vi "Dashboard Main.vi"() -> ()   [LabVIEW 2015]
uses:
  United/Robot Type Def.ctl
  <vilib>/Rock Robotics/WPI/Camera/WPI_CameraWhite Balance Values.ctl
  <vilib>/Rock Robotics/WPI/Camera/WPI_CameraExposure Values.ctl
  <vilib>/Utility/miscctls.llb/LVRowAndColumnTypeDef.ctl
  <vilib>/event_ctls.llb/eventvkey.ctl
  <vilib>/Rock Robotics/WPI/Dashboard/WPI_DashboardLogging Global.vi
  <vilib>/Rock Robotics/Network Tables/NT Read Numeric Array.vi
  <vilib>/Utility/config.llb/Write Key (String).vi
  <vilib>/Utility/config.llb/Write Key (I32).vi
  <vilib>/Utility/config.llb/NI_LVConfig.lvlib
panel:
  in  "5190Settings":refnum<vi>[][](array[refnum])
  in  "TCP":refnum<k5>
  in  "Rec Mode":enum32{"Stop", "Record", "Playback"}(radio)
  in  "Vision":u16(ring) items=["Camera Off", "USB Camera SW", "USB Camera HW", "IP Camera"]
  out "Camera IP":string
  out "Image Message":string="Timeout in Camera Communications"
  in  "Dashboard Tab":T1(tab)
  in  "Select Auto":string(combo)
  out "NT Connection":bool
  in  "Camera Settings":T2={"Frame Rate"=30, "Compression"=30, "Size"=1} {"Frame Rate" scale=1.0..30.0; "Size" items=["640x480", "320x240", "160x120"]}
  out "MotorChart R":cluster{"Numeric":dbl, "Numeric":dbl}(graph)
  out "MotorChart L":T3(graph)
  out "MotorSliders R":cluster{"MotorSlide1":dbl, "MotorSlide2":dbl} {"MotorSlide2" scale=-1.0..1.0 scale format="%#_2e"; "MotorSlide1" scale=-1.0..1.0 scale format="%#_2e"}
  out "MotorSliders L":T4 {"MotorSlide4 2" scale=0.0..14.0 scale format="%#_2e"; "MotorSlide2" scale=-1.0..1.0 scale format="%#_2e"; "MotorSlide1" scale=-1.0..1.0 scale format="%#_2e"}
  out "Gyro":dbl(knob) scale=0.0..360.0
  out "JS1 Z":dbl(slide) scale=-1.0..1.0 scale format="%#_2e"
  out "JS1 Graph":cluster{"X":dbl, "Y":dbl}[](graph)
  out "JS1 Buttons":T5
  out "JS2 Z":dbl(slide) scale=-1.0..1.0 scale format="%#_2e"
  out "JS2 Graph":cluster{"X":dbl, "Y":dbl}[](graph)
  out "JS2 Buttons":T5
  out "Mode":T6(ring)=enum."Auto Disabled"
  in  "DB Camera Config":bool
  out "fps":dbl format="%#.1g"
  out "Mbps":dbl format="%#.1g"
  out "Mbps LED":bool
  in  "Test Slider":dbl(slide) scale=0.0..100.0 scale format="%#_3g"
  in  "On/Off":bool caption="Solenoid"
  in  "Test Name":u16(ring) items=["Select the test to run..."]
  in  "Test Tree":string(tree)
  in  "Motor":cluster{"Value":dbl, "Enable":bool} {"Value" scale=-1.0..1.0 scale format="%#_3g"}
  out "Progress":T7 {"Test Progress" scale=0.0..100.0}
  in  "Rev/Fwd":cluster{"Forward":bool, "Reverse":bool}
  in  "Test Ring":u16(ring) items=["Monochrome", "Color"]
  out "Cmd Status":string
  in  "Execute Command":bool
  in  "Command Params":string[][](table)
  in  "Command Selection":i32(listbox)
  in  "CheckList":i32(listbox)
  out "Tree":string(tree)
  in  "Tab Control":T8(tab)
  in  "Joystick Deadband":dbl format="%#_13g"
  out "Sent":bool
  in  "Send Values to Robot":bool
  in  "Robot":T9
  in  "AutoPlaySelect":T10(ring)=enum."Play02"
  in  "EncTics5":dbl
  in  "updistance":dbl
  in  "Radius":dbl
  in  "R5":dbl
  in  "IZ5":dbl
  in  "F5":dbl
  in  "D5":dbl
  in  "I5":dbl
  in  "P5":dbl
  in  "Turn Damp":dbl format="%#_13g"
  in  "P 2":dbl format="%#_13g"
  in  "I 2":dbl format="%#_13g"
  in  "D 2":dbl format="%#_13g"
  in  "F 2":dbl format="%#_13g"
  in  "R 2":dbl format="%#_13g"
  in  "IZ 2":dbl format="%#_13g"
  in  "P":dbl format="%#_13g"
  in  "I":dbl format="%#_13g"
  in  "D":dbl format="%#_13g"
  in  "R":dbl format="%#_13g"
  in  "F":dbl format="%#_13g"
  in  "IZ":dbl format="%#_13g"
  in  "EncTicsPerRev":dbl format="%#_13g"
  in  "ClimberRevs":dbl
  in  "P 3":dbl format="%#_13g"
  in  "IZ 3":dbl format="%#_13g"
  in  "R 3":dbl format="%#_13g"
  in  "I 3":dbl format="%#_13g"
  in  "F 3":dbl format="%#_13g"
  in  "D 3":dbl format="%#_13g"
  in  "Up Angle(Ticks)":dbl format="%#_13g"
  in  "EncTicsPerRev 2":dbl format="%#_13g"
  in  "Down Angle(Ticks)":dbl format="%#_13g"
  in  "Shoot Delay":dbl
  in  "Shoot Continue":dbl
  in  "Intake Close Claw":dbl
  in  "Intake Time Limit":dbl
  in  "DeltaAngle":dbl
  in  "TopOutSpeed":dbl
  in  "BottomOutSpeed":dbl
  in  "TopInSpeed":dbl
  in  "BottomInSpeed":dbl
  in  "P 4":dbl format="%#_13g"
  in  "IZ 4":dbl format="%#_13g"
  in  "R 4":dbl format="%#_13g"
  in  "I 4":dbl format="%#_13g"
  in  "F 4":dbl format="%#_13g"
  in  "D 4":dbl format="%#_13g"
  in  "EncTicsPerRev 3":dbl format="%#_13g"
  in  "Brightness":dbl
  in  "Compression":dbl
  in  "Exposure":T11=enum."Flicker-free 60 Hz"
  in  "White Balance":T12=enum."Fixed indoor"
  in  "FPS":dbl
  in  "Masked":bool
  in  "LED Color":T13={"Hue"={110.52399131877658, 148.6727294921875}, "Sat"={34.78571428571429, 255.0}, "Val"={91.07142857142858, 255.0}} {"Hue" scale=0.0..255.0 scale format="%#_3g"}
  out "X Deg":dbl
  out "Y Deg":dbl
  in  "LapTop Cam":bool
  out "Camera Image":T14(plugin-control)
  out "Background":bool
  # "Left"
  # "Front"
  # "Right"
  # "Battery"
  # "Autonomous Mode Save File: /home/lvuser/Autonomous/Play/Play##.csv\nCommands:\nTime:\n    0   MS       0      0\n\nStraight:\n    1   INCHES   0      0 \n\nTurn:\n    2   ANGLE    SPEED  0   \n \nArm Set Angle:\n    3   ANGLE    0      0 \n\nShoot:\n    4   0              0            0"
  # "PID for the Tape"
  # "All Units in Inches"
  # "Distance"
  # "Speed"
  # "Postion"
  # "Roller Speeds"
  # "Shooter ARM PID"
  # "Solenoid Delays"
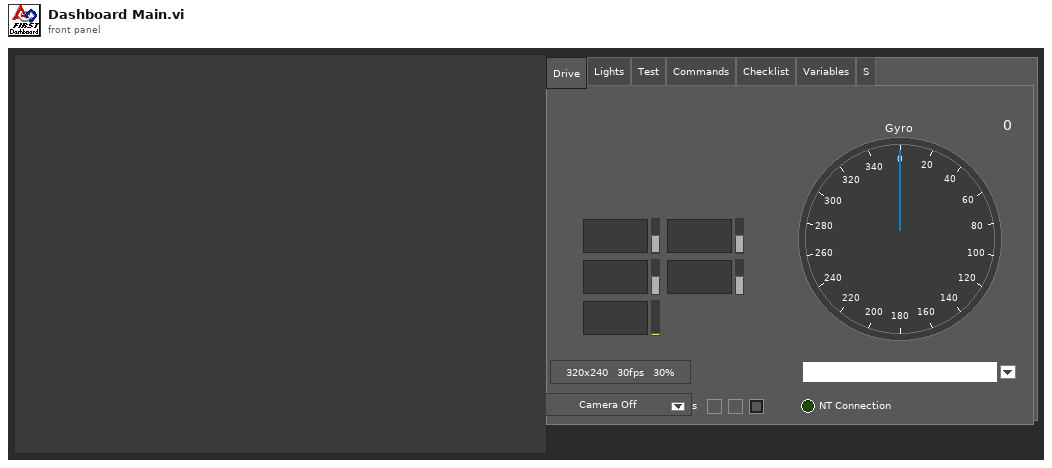
[diagram p1: front panel]
types:
  T1 = enum32{"Drive", "Lights", "Test", "Commands", "Checklist", "Variables", "S"}
  T2 = cluster{"Frame Rate":i32, "Compression":i32, "Size":u16}
  T3 = cluster{"Numeric":dbl, "Numeric":dbl, "Battery V":dbl}
  T4 = cluster{"MotorSlide1":dbl, "MotorSlide2":dbl, "MotorSlide4 2":dbl}
  T5 = cluster{bool, bool, bool, bool, bool, bool, bool, bool, bool, bool, bool, bool}
  T6 = enum8{"Tele-Op Disabled", "Tele-Op Enabled", "Auto Disabled", "Auto Enabled", "Test Disabled", "Test Enabled", "Disconnected", "No Code", "E-Stop"}
  T7 = cluster{"Test Progress":u8, "Test Progress Text":string}
  T8 = enum32{"Main", "Auto", "Tape", "Drive", "Port C", "Shooter", "Vision"}
  T9 = typedef "Robot Type Def.ctl" = enum32{"Disabled", "Ghost", "Casper", "Lofty", "Board", "RaceRobot"}
  T10 = enum16{"Play00", "Play01", "Play02", "Play03", "Play04", "Play05"}
  T11 = typedef "WPI_CameraExposure Values.ctl" = enum16{"Auto", "Flicker-free 50 Hz", "Flicker-free 60 Hz", "Hold current", "Custom"}
  T12 = typedef "WPI_CameraWhite Balance Values.ctl" = enum16{"Auto", "Fixed indoor", "Fixed outdoor 1", "Fixed outdoor 2", "Fixed fluorescent 1", "Fixed fluorescent 2", "Hold current", "Custom"}
  T13 = cluster{"Hue":cluster{dbl, dbl}, "Sat":cluster{dbl, dbl}, "Val":cluster{dbl, dbl}}
  T14 = typedef "IMAQ Image.ctl" = refnum<image>
  T15 = typedef "Image Type" = u32
  T16 = cluster{"IDs":cluster{"RPC field ID":u16, "Unique ID":u16}, "String":string}
  T17 = enum32{"Drive", "Lights", "Test", "Commands", "Checklist", "Variables"}
  T18 = enum32{"Drive", "Basic", "Custom", "Test", "Checklist", "Variables"}
  T19 = cluster{"Camera Image":refnum<vi>, "Dashboard Tab":refnum<vi>, "Background":refnum<vi>, "Vision":refnum<vi>, "Rec Mode":refnum<vi>, "Test Slider":refnum<vi>, "On/Off ":refnum<vi>, "Test Ring":refnum<vi>, "Rev/Fwd":refnum<vi>, "Test Name":refnum<vi>, "Motor":refnum<vi>, "Progress":refnum<vi>, "CheckList":refnum<vi>, "Tree":refnum<vi>, "Test Tree":refnum<vi>, "Command Params":refnum<vi>, "Command Selection":refnum<vi>, "Execute Command":refnum<vi>, "Cmd Status":refnum<vi>}
  T20 = cluster{"Error Strings":string, "Disable Counts":cluster{u16, u16}, "Rail Faults":cluster{u16, u16, u16}, "Robot IP":string, "DB Mode":u8, "Event Info":cluster{"Name":string, "Type":u8, "Number":u16, "Replay":u8}, "Camera Addr":string}
  T21 = cluster{"Storage":cluster{"Disk Free":u64, "RAM Block":u32, "RAM free":u32}, "CPU Utilization":cluster{"CPU % ISR":sgl, "CPU % Time Crit":sgl, "CPU % Timed Str":sgl, "CPU % High":sgl, "CPU % Above":sgl, "CPU % Normal":sgl, "CPU % Low":sgl}, "CAN":cluster{"% Bus Utilization":sgl, "Bus Off Cnt":u32, "TX_FIFO Full Cnt":u32, "Receive Error Cnt":u8, "Transmit Error Cnt":u8}, "HID":cluster{"HID Outputs":u32, "Rumble Low":u16, "Rumble High":u16}[]}
  T22 = cluster{"Status bits":cluster{"Test Mode":bool, "Autonomous":bool, "Enabled":bool, "Code Start":bool, "Brownout":bool, "Reserved 2":bool, "Reserved 3":bool, "E-Stop":bool}, "Code Trace":cluster{"Disabled":bool, "TeleOp":bool, "Auto":bool, "Test":bool}, "Controller Type":enum16{"unknown", "cRIO", "roboRio"}, "Code?":enum16{"unknown", "noCode", "code"}, "Battery V":dbl}
  T23 = cluster{"Control Bits":cluster{"TestMode":bool, "Autonomous":bool, "Enabled":bool, "FMS Present":bool, bool, bool, bool, "E-Stop":bool}, "Team Station ":u8, "Countdown":sgl, "Joystick Values":cluster{"Axes":dbl[], "Buttons":bool[], "POVs":i16[]}[]}
  T24 = cluster{"Axes":dbl[], "Buttons":bool[], "POVs":i16[]}[]
  T25 = cluster{"Axes":dbl[], "Buttons":bool[], "POVs":i16[]}
  T26 = cluster{"Buttons[0]":bool, "Buttons[1]":bool, "Buttons[2]":bool, "Buttons[3]":bool, "Buttons[4]":bool, "Buttons[5]":bool, "Buttons[6]":bool, "Buttons[7]":bool, "Buttons[8]":bool, "Buttons[9]":bool, "Buttons[10]":bool, "Buttons[11]":bool}
  T27 = typedef "NI_LVConfig.lvlib/Config Data RefNum.ctl" = refnum<k1>
  T28 = cluster{"Operation":enum16{"Update", "Clear"}, "Color Box":u32}[]
  T29 = typedef "eventvkey.ctl" = enum16{"ASCII", "Enter", "Return", "Shift", "Ctrl", "Alt", "Cmd", "Opt", "Caps", "NumLock", "Clear", "Break", "Up", "Down", "Left", "Right", "Insert", "Delete", "Home", "End", "PageUp", "PageDown", "Escape", "Help", "Pause", "ScrollLock", "F1", "F2", "F3", "F4", "F5", "F6", "F7", "F8", "F9", "F10", "F11", "F12", "F13", "F14", "F15", "F16", "F17", "F18", "F19", "F20", "F21", "F22", "F23", "F24", "Play", "VolumeUp", "VolumeDown", "Mute", "Two Byte Char"}
  T30 = cluster{"Image Size":bool, "Image Type":bool, "Pixel Value":bool, "ROI Information":bool, "Zoom Factor":bool}
  T31 = enum8{"Enabled", "Disabled", "Disabled and Grayed Out"}
  T32 = cluster{"Operation":enum16{"Update", "Clear"}, "Color Box":u32}
  T33 = typedef "LVRowAndColumnTypeDef.ctl" = cluster{"Row":i32, "Column":i32}
  T34 = cluster{"Shift":bool, "Ctrl":bool, "Alt":bool, "Cmd":bool, "Opt":bool}
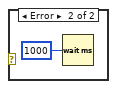
[diagram p2: hidden frame]
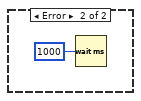
[diagram p3: hidden frame]
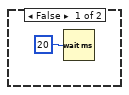
[diagram p4: hidden frame]
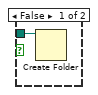
[diagram p6: hidden frame]
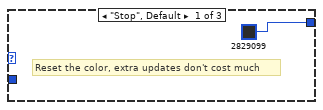
[diagram p7: hidden frame]
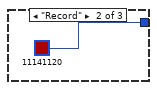
[diagram p8: hidden frame]
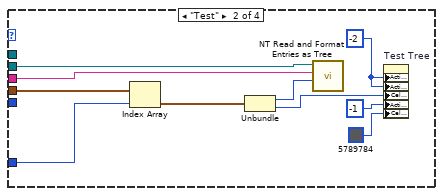
[diagram p10: hidden frame]
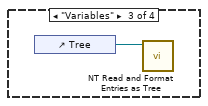
[diagram p11: hidden frame]
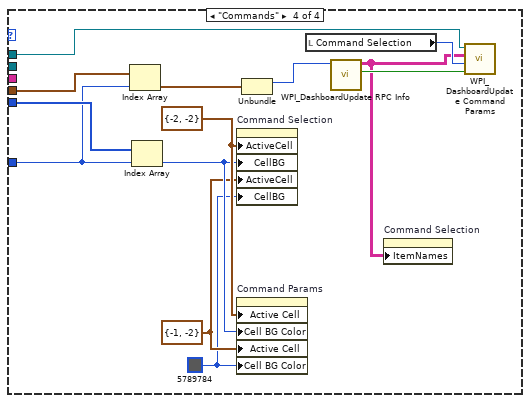
[diagram p12: hidden frame]
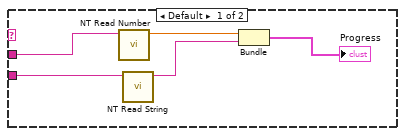
[diagram p13: hidden frame]
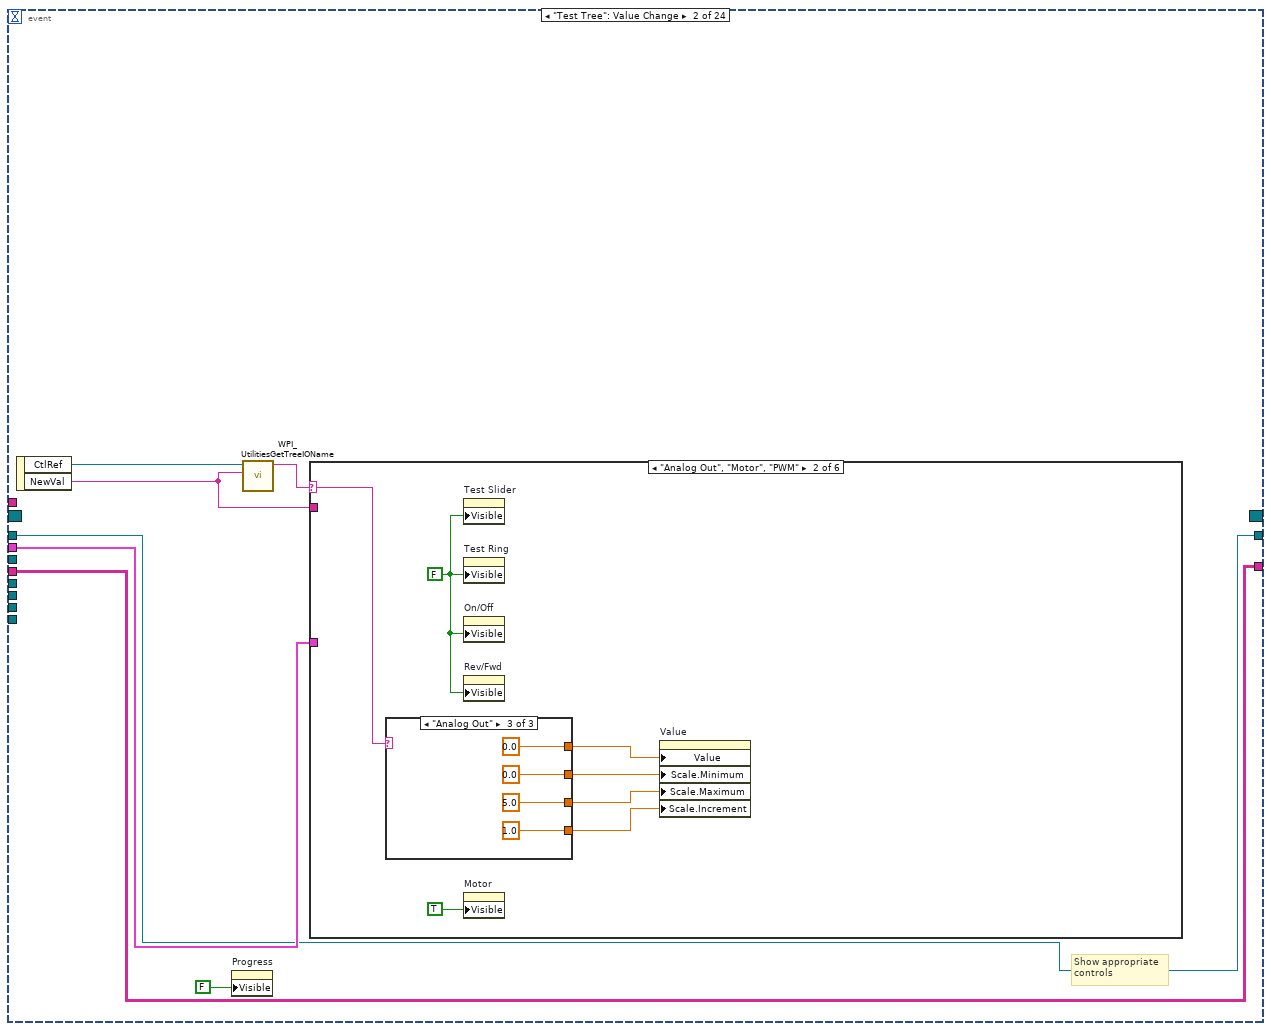
[diagram p14: hidden frame]
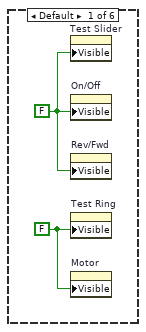
[diagram p15: hidden frame]
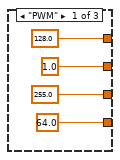
[diagram p16: hidden frame]
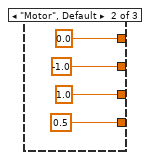
[diagram p17: hidden frame]
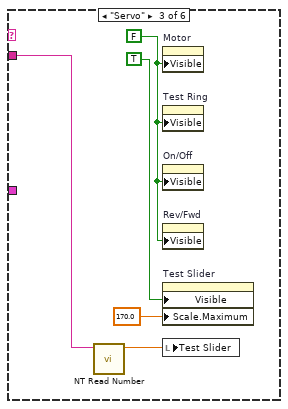
[diagram p18: hidden frame]
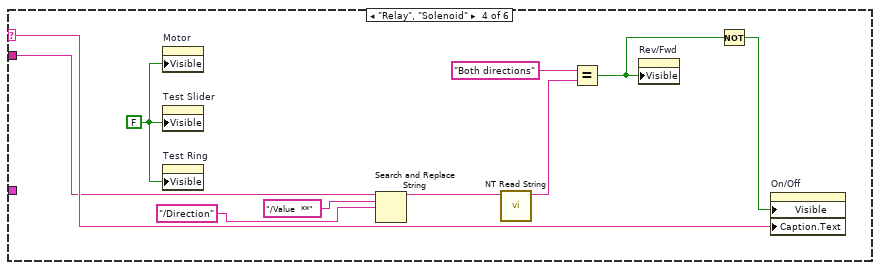
[diagram p19: hidden frame]
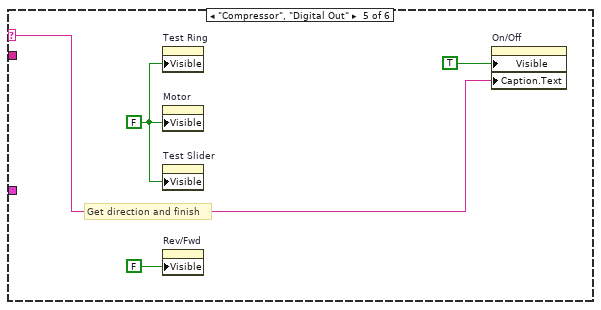
[diagram p20: hidden frame]
diagram:
  w67 = T15 4 items=["Grayscale (U8)", "Grayscale (I16)", "Grayscale (SGL)", "Complex (CSG)", "RGB (U32)", "HSL (U32)", "RGB (U64)", "Grayscale (U16)"] ("Image Type")
  w75 = T16 {"IDs"={"RPC field ID"=0, "Unique ID"=0}, "String"=""}  # RPC Response
  w100 = 491  # min tab size
  w99 = 1.333  # min tab size
  w108 = enum32{"Stop", "Record", "Playback"}."Stop" ("Rec Mode")
  w82 = FALSE ("Visible")
  w128 = T15 4 items=["Grayscale (U8)", "Grayscale (I16)", "Grayscale (SGL)", "Complex (CSG)", "RGB (U32)", "HSL (U32)", "RGB (U64)"] ("Image Type")
  # "Low Shooter\nIndex 3"
  # "Tape \nIndex 5"
  # "Ghost uses Durations and Speeds for In/Out\nCasper uses switches for that"
  # "PortC\nIndex 2"
  # "DriveTrain\nIndex-1"
  # "Robot Type and AutoPlay\nIndex 0"
  # "S"
  # "Open file and read it Once and Only Once"
  # "Command Param Info"
  # "Started one, Unique ID holds\nresponse"
  # "Loop 7. Wait for DS connections"
  # "Basic debug and auto controls: Their data names are fixed, but\nthe displayed name, called a caption, can be changed directly or in\nrobot code such as shown in Begin."
  # "Controls for Test Mode, Camera Settings, etc."
  # "Additional UI Initialization"
  # "Loop 6. Animation for background of window during playback and record"
  # "Fires each time robot IP\nchanges, simulator does this"
  # "Fires each time window\ndocking changes."
  # "Collects all controls and indicators\nin the Basic and Custom tab.\nIf you need to bind additional controls,\nadd their references. You can extend the\nenum constant or use an integer."
  # "The remaining code below this line typically doesn't need to be modified."
  # "Loop 4. Process UI events related to test mode, checklist, and camera settings"
  # "Terminals of controls and indicators that are bound to the smart dashboard by name.\nYou can place the terminals anywhere you like and even read data from them.\nYou bind controls by adding the control reference to the array on the left. The subVI will\ndo this for the contents of a tab, and you can do it for individual items too, as shown with\nthe LED. To create get the reference, right-click and Create>>Reference."
  # "Loop 3. Wait until the robot response provides\n the Robot IP address.\nOnce known, bind controls and\nvariables with the same names."
  # "Loop 5. Adjusts placement onscreen, hides the titlebar, etc."
  # "Loop 2. Receive camera images from Robot, update Mbps, fps, and do any processing or display"
  n1 = control-ref of="DeltaAngle"() -> (w64:refnum<vi>)
  n2 = control-ref of="Joystick Deadband"() -> (w1:refnum<vi>)
  n3 = control-ref of="Robot"() -> (w41:refnum<vi>)
  n4 = control-ref of="updistance"() -> (w23:refnum<vi>)
  n5 = control-ref of="BottomOutSpeed"() -> (w54:refnum<vi>)
  n6 = control-ref of="Intake Time Limit"() -> (w21:refnum<vi>)
  n7 = control-ref of="Intake Close Claw"() -> (w20:refnum<vi>)
  n8 = control-ref of="Up Angle(Ticks)"() -> (w4:refnum<vi>)
  n9 = control-ref of="EncTicsPerRev 3"() -> (w63:refnum<vi>)
  n10 = control-ref of="EncTicsPerRev 2"() -> (w3:refnum<vi>)
  n11 = control-ref of="BottomInSpeed"() -> (w52:refnum<vi>)
  n12 = control-ref of="Shoot Continue"() -> (w18:refnum<vi>)
  n13 = control-ref of="AutoPlaySelect"() -> (w42:refnum<vi>)
  n14 = control-ref of="TopOutSpeed"() -> (w55:refnum<vi>)
  n15 = control-ref of="Down Angle(Ticks)"() -> (w2:refnum<vi>)
  n16 = control-ref of="TopInSpeed"() -> (w53:refnum<vi>)
  n17 = control-ref of="Shoot Delay"() -> (w19:refnum<vi>)
  n18 = control-ref of="P 3"() -> (w10:refnum<vi>)
  n19 = control-ref of="I 3"() -> (w9:refnum<vi>)
  n20 = control-ref of="D 3"() -> (w8:refnum<vi>)
  n21 = control-ref of="F 3"() -> (w7:refnum<vi>)
  n22 = control-ref of="IZ 3"() -> (w6:refnum<vi>)
  n23 = control-ref of="R 3"() -> (w5:refnum<vi>)
  n24 = control-ref of="Brightness"() -> (w12:refnum<vi>)
  n25 = control-ref of="Compression"() -> (w13:refnum<vi>)
  n26 = control-ref of="EncTicsPerRev"() -> (w40:refnum<vi>)
  n27 = control-ref of="Exposure"() -> (w14:refnum<vi>)
  n28 = control-ref of="FPS"() -> (w16:refnum<vi>)
  n29 = control-ref of="ClimberRevs"() -> (w48:refnum<vi>)
  n30 = control-ref of="White Balance"() -> (w15:refnum<vi>)
  n31 = control-ref of="Turn Damp"() -> (w32:refnum<vi>)
  n32 = control-ref of="F 2"() -> (w45:refnum<vi>)
  n33 = control-ref of="IZ 2"() -> (w46:refnum<vi>)
  n34 = control-ref of="R 2"() -> (w47:refnum<vi>)
  n35 = Build Array(w10, w9, w8, w7, w6, w5, w3, w2, w4) -> (w58:refnum<vi>[])
  n36 = control-ref of="P"() -> (w33:refnum<vi>)
  n37 = control-ref of="I"() -> (w34:refnum<vi>)
  n38 = control-ref of="D"() -> (w35:refnum<vi>)
  n39 = control-ref of="F"() -> (w36:refnum<vi>)
  n40 = control-ref of="IZ"() -> (w43:refnum<vi>)
  n41 = control-ref of="R"() -> (w44:refnum<vi>)
  n42 = control-ref of="P 2"() -> (w37:refnum<vi>)
  n43 = control-ref of="I 2"() -> (w38:refnum<vi>)
  n44 = control-ref of="D 2"() -> (w39:refnum<vi>)
  n45 = control-ref of="P 4"() -> (w49:refnum<vi>)
  n46 = control-ref of="I 4"() -> (w50:refnum<vi>)
  n47 = control-ref of="D 4"() -> (w51:refnum<vi>)
  n48 = control-ref of="F 4"() -> (w60:refnum<vi>)
  n49 = control-ref of="IZ 4"() -> (w61:refnum<vi>)
  n50 = control-ref of="R 4"() -> (w62:refnum<vi>)
  n51 = control-ref of="P5"() -> (w31:refnum<vi>)
  n52 = control-ref of="I5"() -> (w30:refnum<vi>)
  n53 = control-ref of="D5"() -> (w29:refnum<vi>)
  n54 = control-ref of="F5"() -> (w28:refnum<vi>)
  n55 = control-ref of="IZ5"() -> (w27:refnum<vi>)
  n56 = control-ref of="R5"() -> (w26:refnum<vi>)
  n57 = control-ref of="EncTics5"() -> (w25:refnum<vi>)
  n58 = control-ref of="Radius"() -> (w24:refnum<vi>)
  n59 = Build Array(w41, w42, w1) -> (w56:refnum<vi>[])
  n60 = Build Array(w33, w34, w35, w36, w43, w44, w37, w38, w39, w45, w46, w47, w40, w48, w32) -> (w57:refnum<vi>[])
  n61 = Build Array(w49, w50, w51, w60, w61, w62, w63, w52, w53, w54, w55, w64, w21, w20, w19, w18) -> (w59:refnum<vi>[])
  n62 = Build Array(w31, w30, w29, w28, w27, w26, w25, w24, w23) -> (w22:refnum<vi>[])
  n63 = Build Array(w16, w15, w14, w13, w12) -> (w11:refnum<vi>[])
  n64 = Build Array(w56, w57, w58, w59, w22, w11) -> (w17:refnum<vi>[][])
  n65 = local write "5190Settings"(w17) -> ()
  n66 = call "Init.vi"("Array"=w17) -> ()  [unwired: 11 in]
  n67 = Obtain Notifier(name (unnamed)="Robot IP Update", notification data type="IP Addr" ("name (unnamed)")) -> (notifier out=w68:refnum<notifier>)  [unwired: 2 in, 2 out]
  n68 = control-ref of="Rec Mode"() -> (w88:refnum<vi>)
  n69 = control-ref of="Command Selection"() -> (w74:refnum<vi>)
  n70 = control-ref of="Camera Image"() -> (w103:refnum<vi>)
  n71 = control-ref of="Tree"() -> (w92:refnum<vi>)
  n72 = control-ref of="Test Tree"() -> (w91:refnum<vi>)
  n73 = control-ref of="Dashboard Tab"() -> (w102:refnum<vi>)
  n74 = control-ref of="Execute Command"() -> (w76:refnum<vi>)
  n75 = control-ref of="Background"() -> (w97:refnum<vi>)
  n76 = control-ref of="On/Off"() -> (w86:refnum<vi>)
  n77 = control-ref of="Progress"() -> (w83:refnum<vi>)
  n78 = control-ref of="Rev/Fwd"() -> (w84:refnum<vi>)
  n79 = control-ref of="Motor"() -> (w89:refnum<vi>)
  n80 = control-ref of="Cmd Status"() -> (w70:refnum<vi>)
  n81 = control-ref of="Command Params"() -> (w77:refnum<vi>)
  n82 = control-ref of="Test Slider"() -> (w87:refnum<vi>)
  n83 = control-ref of="Vision"() -> (w101:refnum<vi>)
  n84 = control-ref of="Test Ring"() -> (w85:refnum<vi>)
  n85 = control-ref of="Test Name"() -> (w90:refnum<vi>)
  n86 = property class="VI" props=["Front Panel.Closeable"]() -> (reference out=w107:refnum<vi>)  [unwired: 2 in, 2 out]
  n87 = control-ref of="Command Params"() -> (w69:refnum<vi>)
  n88 = control-ref of="CheckList"() -> (w93:refnum<vi>)
  n89 = Bundle("min tab size"=w100, "min tab size"=w99) -> (w98:cluster{"min tab size":i32, "min tab size":dbl})  [unwired: 1 in]
  n90 = Create User Event(user event datatype=w75) -> (user event=w71:refnum<user-event>)  [unwired: 1 in, 1 out]
  n91 = Obtain Notifier(name (unnamed)="Window Mode", notification data type=TRUE) -> (notifier out=w80:refnum<notifier>)  [unwired: 2 in, 2 out]
  n92 = Bundle("Camera Image"=w103, "Dashboard Tab"=w102, "Background"=w97, "Vision"=w101, "Rec Mode"=w88, "Test Slider"=w87, "On/Off"=w86, "Test Ring"=w85, "Rev/Fwd"=w84, "Test Name"=w90, "Motor"=w89, "Progress"=w83, "CheckList"=w93, "Tree"=w92, "Test Tree"=w91, "Command Params"=w77, "Command Selection"=w74, "Execute Command"=w76, "Cmd Status"=w70) -> (w94:T19)  [unwired: 1 in]
  n93 = control-ref of="Dashboard Tab"() -> (w106:refnum<vi>)
  n94 = call "IMAQ Create"("Image Name"="Dashboard Image", "Image Type"=w128) -> ("New Image"=w126:T14, "error out"=w125:errorcluster)  [unwired: 2 in, 1 out]
  n95 = call "IMAQ Create"("Image Name"="LapTop Cam", "Image Type"=w67) -> ("New Image"=w65:T14)  [unwired: 2 in, 2 out]
  n96 = call <vilib>:"Get Tab Control Refs.vi"("Page Index"=T18."Basic" ("Dashboard Tab"), "TabControl in"=w106) -> ("ControlsOnPage"=w81:refnum<vi>[])  [unwired: 9 in]
  n97 = while {
    tunnel: [w142] -> _
    tunnel: w68 -> [w137]
    tunnel: w81 -> [w136]
    tunnel: w80 -> [w132]
    i -> [w142]
    stop <- FALSE stop-if-true
    n98 = call <vilib>:"WPI_DashboardUpdateNames.vi"("Controls on Tab"=w136) -> ()  [unwired: 11 in]
    n99 = local read "Vision"() -> (w134:u16)
    n100 = call <vilib>:"WPI_DashboardRetrieveStatusInfo.vi"("Vision"=w134, "Binding Refnum"=w137, "Window Mode Notifier"=w132, "TCP Cnx"="TCP") -> ("Power and Errors"=w138:T20, "Robot Metrics"=w140:T21, "Status Info"=w141:T22, "Control Info"=w139:T23, "Robot Mode"=w135:T6, "Process?"=w131:bool)  [unwired: 2 in]
    "Mode" <- w135
    n101 = feedback-in #1(w131) -> ()
    n102 = feedback #1(FALSE) -> (w129:bool)
    n103 = case shown="True" w131 {
      tunnel: w141 -> [_ w175]
      tunnel: w140 -> [_ w174]
      tunnel: w139 -> [_ w173]
      tunnel: w138 -> [_ w172]
      tunnel: w135 -> [_ _]
      tunnel: w129 -> [_ w148]
      frame False {
        n104 = Wait (ms)(milliseconds to wait=u32 20) -> ()  [unwired: 1 out]
      }
      frame True {
        # "swap motors to match\ncharts and include battery"
        n105 = Not(x=w148) -> (.not. x?=w146:bool)
        n106 = Unbundle By Name(w173) -> ("Joystick Values"=w162:T24)  [unwired: 1 out]
        n107 = Unbundle By Name(w174) -> ()  [unwired: 1 out]
        n108 = Unbundle By Name(w172) -> ("Camera Addr"=→"Camera IP":string)  [unwired: 1 out]
        n109 = Unbundle By Name(w175) -> ("Battery V"=w163:dbl)  [unwired: 1 out]
        n110 = Or(x="Send Values to Robot", y=w146) -> (x .or. y?=w145:bool)
        n111 = Index Array(array=w162) -> (element #1=w161:T25, element #2=w156:T25)  [unwired: 2 in]
        n112 = case shown="True" w145 {
          frame False {
          }
          frame True {
            n113 = flat-sequence {
              tunnel: [TRUE] -> w176
              frame #0 {
                n114 = local write "Sent"(FALSE) -> ()
              }
              frame #1 {
                w178 = path "C:/5190data" ("path")
                n115 = call <vilib>:"Check if File or Folder Exists.vi"("path"=w178) -> ("file or folder exists?"=w179:bool)  [unwired: 8 in, 2 out]
                n116 = case shown="True" w179 {
                  tunnel: w178 -> [w180 _]
                  frame False {
                    n117 = Create Folder(path (use dialog)=w180) -> ()  [unwired: 2 in, 3 out]
                  }
                  frame True {
                  }
                }
              }
              frame #2 {
                n118 = local read "5190Settings"() -> (w182:refnum<vi>[][])
                n119 = call "Read-Write-Settings.vi"("appended array 4"=w182, "Write"=TRUE) -> ()  [unwired: 5 in, 1 out]
              }
            }
            "Sent" <- w176
          }
        }
        n120 = call-poly <vilib>:"NT Read Value.vi"("Name"="NavX Yaw") -> ("Numeric"=→"Gyro":dbl)  [unwired: 9 in, 1 out]
        n121 = call "Prepare Joystick Data for Displays.vi"("Joystick Values"=w161) -> ("Buttons"=→"JS1 Buttons":T26, "Z Axis"=→"JS1 Z":dbl, "Cartesian Data"=→"JS1 Graph":cluster{"X axis":dbl, "X axis":dbl}[])  [unwired: 8 in]
        n122 = call "Prepare Joystick Data for Displays.vi"("Joystick Values"=w156) -> ("Buttons"=→"JS2 Buttons":T26, "Z Axis"=→"JS2 Z":dbl, "Cartesian Data"=→"JS2 Graph":cluster{"X axis":dbl, "X axis":dbl}[])  [unwired: 8 in]
        n123 = call-poly <vilib>:"NT Read Value.vi"("Name"="RobotDrive Motors") -> ("Numeric Array"=w151:dbl[])  [unwired: 9 in, 1 out]
        n124 = Index Array(array=w151, index #1=1, index #4=0) -> (element #1=w167:dbl, element #2=w168:dbl, element #3=w166:dbl, element #4=w171:dbl)  [unwired: 2 in]
        n125 = Bundle("Numeric"=w166, "Numeric"=w167) -> (→"MotorChart R" →"MotorSliders R":cluster{"Numeric":dbl, "Numeric":dbl})  [unwired: 1 in]
        n126 = Bundle("Numeric"=w168, "Numeric"=w171, "Battery V"=w163) -> (→"MotorChart L" →"MotorSliders L":T3)  [unwired: 1 in]
      }
    }
  }
  n127 = call <vilib>:"Get Tab Control Refs.vi"("Page Index"=T18."Custom" ("Dashboard Tab"), "TabControl in"=w106) -> ("ControlsOnPage"=w105:refnum<vi>[])  [unwired: 9 in]
  n128 = while {
    tunnel: w126 -> [w199]
    tunnel: w125 -> [_]
    tunnel: [w200] -> _
    tunnel: w65 -> [w197]
    i -> [w200]
    stop <- FALSE stop-if-true
    n129 = local read "Camera IP"() -> (w195:string)
    n130 = local read "Rec Mode"() -> (w192:enum32{"Stop", "Record", "Playback"})
    n131 = call "Untitled 3 (SubVI).vi"("Refnum in"=w197, "LapTop Cam"="LapTop Cam", "Vision"="Vision", "New Image in"=w199, "Camera IP"=w195, "Rec Mode"=w192, "Show Black And White"="Masked", "LED Color"="LED Color", "Camera Settings"="Camera Settings") -> ("Bandwidth (Mbps)"=→"Mbps":dbl, "Refnum out"=→"Camera Image":T14, "Array"=w190:cluster{"Color Box":u32, "Color Box":u32}[], "Numeric 2"=→"X Deg":dbl, "Numeric"=→"Y Deg":dbl, "FPS"=→"fps":dbl, "status"=w186:bool)
    n132 = property on="Mbps LED" class="Bool (strict)"("Colors [4]"=w190) -> ()  [unwired: 2 in, 2 out]
    n133 = property on="Image Message" class="Str"("Visible"=w186) -> ()  [unwired: 2 in, 2 out]
  }
  n134 = Build Array (concatenate)(w81, w105) -> (w104:refnum<vi>[])
  n135 = call "Adjust Dashboard Window.vi"("Sizing Refnums"=w94, "Size Constraints"=w98, "VI"=w107, "WIn Mode"=w80) -> ()  [unwired: 8 in]
  n136 = register-events(refnum<vi> refnum, w71) -> (reference out=w112:refnum<event-registration>, error out=w111:errorcluster)  [unwired: 2 in]
  n137 = property class="VI"() -> ("Panel"=w115:refnum<vi>)  [unwired: 2 in, 2 out]
  n138 = while {
    tunnel: w104 -> [w214]
    tunnel: w68 -> [w212]
    tunnel: [w210] -> _
    tunnel: u32 1000 ("milliseconds to wait") -> [w209]
    tunnel: w71 -> [w202]
    i -> [w210]
    stop <- FALSE stop-if-true
    n139 = local read "Rec Mode"() -> (w205:enum32{"Stop", "Record", "Playback"})
    n140 = Wait on Notification(notifier=w212, timeout in ms (-1)=w209) -> (notification=w211:string, timed out?=w207:bool)  [unwired: 2 in, 2 out]
    n141 = Equal?(x=w205, y=u16 2 ("Rec Mode")) -> (x = y?=w206:bool)
    n142 = Compound Arithmetic op=OR(invert w207, w206) -> (w208:bool)
    n143 = case shown="True" w208 {
      tunnel: w214 -> [_ w218]
      tunnel: w211 -> [_ w217]
      tunnel: "Dashboard" -> [_ w216]
      tunnel: w202 -> [_ w215]
      frame False {
      }
      frame True {
        n144 = call <vilib>:"Bind Controls to SmartDashboard.vi"("RPC ref"=w215, "Client Name"=w216, "Bound Control Refs"=w218, "Server IP Address"=w217) -> ()  [unwired: 8 in]
      }
    }
  }
  n145 = vi-ref "Playback Controls.vi"() -> (w113:refnum<vi>)
  n146 = call "Initialize Camera and CheckList.vi"("ListBox in"=w93) -> ("Cluster"=w119:cluster{"value":i32, "value":i32, "index":i32}, "Array"=w120:cluster{string[]}[], "File Refnum"=w118:T27)  [unwired: 8 in]
  n147 = property class="Pnl"(reference=w115) -> ("Panes[]"=w116:refnum<vi>[])  [unwired: 1 in, 2 out]
  n148 = property on="Camera Settings" class="Clust (strict)"("Val(Sgnl)"=w119) -> ()  [unwired: 2 in, 2 out]
  n149 = Index Array(array=w116) -> (element=w114:refnum<vi>)  [unwired: 1 in]
  n150 = control-ref of="Test Tree"() -> (w117:refnum<vi>)
  n151 = while {
    tunnel: w120 -> [w230]
    shift-right: [w229] -> _
    shift-left: w118 -> [w228]
    tunnel: [w227] -> _
    tunnel: w117 -> [w226]
    tunnel: w113 -> [w225]
    tunnel: w112 -> [w224]
    tunnel: w111 -> [_]
    tunnel: w107 -> [w223]
    tunnel: w71 -> [w222]
    tunnel: w69 -> [w221]
    shift-right: [w220] -> _
    shift-left: _ -> [w219]
    i -> [w227]
    stop <- FALSE stop-if-true
    n152 = event shown="[0] Timeout" {
      selector: w224 -> [_ _ _ _ _ _ _ _ _ _ _ _ _ _ _ _ _ _ _ _ _ _ _ _]
      dyn-events: [_ _ _ _ _ _ _ _ _ _ _ _ _ _ _ _ _ _ w539 _ _ _ _ _] -> _
      timeout: u32 60 ("milliseconds to wait") -> [_ _ _ _ _ _ _ _ _ _ _ _ _ _ _ _ _ _ _ _ _ _ _ _]
      tunnel: w226 -> [w243 _ _ _ _ _ _ _ _ _ _ _ _ _ _ _ _ _ _ _ _ _ _ _]
      tunnel: "Test Tree" -> [_ _ _ _ _ _ _ _ _ _ _ _ _ w502 w511 w514 w519 w528 _ _ _ _ _ _]
      tunnel: w230 -> [_ w281 _ _ _ _ _ _ _ _ _ w464 w495 _ _ _ _ _ _ _ _ _ _ _]
      tunnel: [w240 w280 w384 w390 w400 w404 w410 w422 w430 w436 w449 w463 w488 w501 w509 w513 w518 w527 w541 w557 w559 w567 w578 w583] -> w229
      tunnel: w228 -> [w240 w280 w384 w390 w400 w404 w410 w422 w430 w436 w449 w462 w488 w501 w509 w513 w518 w527 w541 w557 w559 w567 w578 w583]
      tunnel: w225 -> [_ _ _ _ _ _ _ _ _ _ _ _ _ _ _ _ _ _ w542 _ w562 _ _ _]
      tunnel: w223 -> [_ _ _ _ _ _ _ _ _ _ _ _ _ _ _ _ _ _ w537 _ _ _ _ _]
      tunnel: w222 -> [_ _ _ _ _ _ _ _ _ _ _ _ _ _ _ _ _ _ w533 _ _ _ _ _]
      tunnel: w221 -> [w235 _ _ _ _ _ w408 _ _ _ _ _ _ _ _ _ _ _ _ _ _ _ _ _]
      tunnel: [w234 w279 w383 w389 w399 w405 w406 w416 w427 w435 w448 w461 w487 w500 w508 w512 w517 w526 w532 w555 w558 w563 w571 w584] -> w220
      tunnel: w219 -> [w234 w279 w383 w389 w399 w405 w406 _ _ w435 w448 w461 w487 w500 w508 w512 w517 w526 w532 w555 w558 w563 w571 w584]
      event Timeout {
        n153 = event-data() -> ()  [unwired: 1 in, 1 out]
        n154 = call <vilib>:"Connextion Info.vi"() -> ("Connected"=→"NT Connection":bool)  [unwired: 10 in, 1 out]
        n155 = call <vilib>:"NT Read String.vi"("Name"="/TestMode/TestName") -> ("String"=w246:string)  [unwired: 9 in, 1 out]
        n156 = case shown="\"\"" w246 {
          tunnel: "/TestMode/TestProgress" ("Name") -> [w273 _]
          tunnel: "/TestMode/TestProgressText" ("Name") -> [w272 _]
          frame Default {
            n157 = call <vilib>:"NT Read Number.vi"("Name"=w273) -> ("Numeric"=w274:dbl)  [unwired: 9 in, 1 out]
            n158 = call <vilib>:"NT Read String.vi"("Name"=w272) -> ("String"=w275:string)  [unwired: 9 in, 1 out]
            n159 = Bundle("Numeric"=w274, "String"=w275) -> (→"Progress":cluster{"Numeric":dbl, "String":string})  [unwired: 1 in]
          }
          frame "" {
            n160 = local write "Test Name"(u16 0) -> ()
            n161 = property on="Progress" class="Clust (strict)"("Visible"=FALSE) -> ()  [unwired: 2 in, 2 out]
          }
        }
        n162 = local read "Mode"() -> (w237:T6)
        n163 = case shown="\"Lights\", \"S\", Default" "Dashboard Tab" {
          tunnel: w243 -> [_ w257 _ _]
          tunnel: "/TestMode/Automatic/" ("Name Pattern") -> [_ w256 _ _]
          tunnel: T28 [{"Operation"=enum."Clear", "Color Box"=14013909}, {"Operation"=enum."Clear", "Color Box"=14013909}, {"Operation"=enum."Clear", "Color Box"=14013909}, {"Operation"=enum."Clear", "Color Box"=14013909}, {"Operation"=enum."Update", "Color Box"=14013909}, {"Operation"=enum."Update", "Color Box"=16777215}, {"Operation"=enum."Clear", "Color Box"=14013909}, {"Operation"=enum."Clear", "Color Box"=14013909}, {"Operation"=enum."Clear", "Color Box"=14013909}] -> [_ w249 _ w266]
          tunnel: w237 -> [_ w248 _ w265]
          tunnel: u32[] [15790320, 15790320, 15790320, 15790320, 16777215, 16777215, 15790320, 15790320, 15790320] -> [_ _ _ w271]
          tunnel: w235 -> [_ _ _ w259]
          frame "Lights", "S", Default {
          }
          frame "Test" {
            w255 = -2 ("Active Item:Row Number")
            n164 = Index Array(array=w249, index=w248) -> (element=w250:T32)
            n165 = Unbundle(w250) -> ("Operation"=w251:enum16{"Update", "Clear"}, "Color Box"=w252:u32)
            n166 = call <vilib>:"NT Read and Format Entries as Tree.vi"("Operation"=w251, "Name Pattern"=w256, "Tree Refnum"=w257) -> ()  [unwired: 7 in, 2 out]
            n167 = property on="Test Tree" class="Tree (strict)"("Active Item Row Number"=w255, "ActiveColNum"=w255, "CellBG"=w252, "Active Item Row Number"=-1 ("Active Item:Row Number"), "CellBG"=u32 5789784 ("Color Box")) -> ()  [unwired: 2 in, 2 out]
          }
          frame "Variables" {
            n168 = control-ref of="Tree"() -> (w258:refnum<vi>)
            n169 = call <vilib>:"NT Read and Format Entries as Tree.vi"("Tree Refnum"=w258) -> ()  [unwired: 9 in, 2 out]
          }
          frame "Commands" {
            w267 = u32 5789784 ("Color Box")
            w268 = T33 {"Row"=-1, "Column"=-2} ("Active Cell:Active Cell")
            w270 = T33 {"Row"=-2, "Column"=-2} ("Active Cell:Active Cell")
            n170 = Index Array(array=w266, index=w265) -> (element=w264:T32)
            n171 = Index Array(array=w271, index=w265) -> (element=w269:u32)
            n172 = property on="Command Selection" class="MCListbox (strict)"("ActiveCell"=w270, "CellBG"=w269, "ActiveCell"=w268, "CellBG"=w267) -> ()  [unwired: 2 in, 2 out]
            n173 = property on="Command Params" class="Tbl (strict)"("Active Cell"=w270, "Cell BG Color"=w269, "Active Cell"=w268, "Cell BG Color"=w267) -> ()  [unwired: 2 in, 2 out]
            n174 = Unbundle(w264) -> ("Operation"=w263:enum16{"Update", "Clear"})  [unwired: 1 out]
            n175 = local read "Command Selection"() -> (w262:i32)
            n176 = call <vilib>:"WPI_DashboardUpdate RPC Info.vi"("Operation"=w263) -> ("update"=w261:bool, "commands"=w260:string[][])  [unwired: 9 in]
            n177 = property on="Command Selection" class="MCListbox (strict)"("ItemNames"=w260) -> ()  [unwired: 2 in, 2 out]
            n178 = call <vilib>:"WPI_DashboardUpdate Command Params.vi"("Update"=w261, "NewVal"=w262, "Commands"=w260, "Param Tbl"=w259) -> ()  [unwired: 7 in, 1 out]
          }
        }
      }
      event "Test Tree": Value Change {
        # "Show appropriate\ncontrols"
        n179 = event-data() -> ("CtlRef"=w284:refnum<vi>, "NewVal"=w282:string)  [unwired: 1 in]
        n180 = property on="Progress" class="Clust (strict)"("Visible"=FALSE) -> ()  [unwired: 2 in, 2 out]
        n181 = call <vilib>:"WPI_UtilitiesGetTreeIOName.vi"("NewVal"=w282, "TreeControl in"=w284) -> ("I/O Name"=w285:string)  [unwired: 9 in]
        n182 = case shown="\"Analog Out\", \"Motor\", \"PWM\"" w285 {
          selector: w285 -> [_ w292 _ w314 w323 _]
          tunnel: w282 -> [_ _ w311 w313 _ w330]
          tunnel: w281 -> [_ _ _ _ _ w329]
          frame Default {
            w287 = FALSE ("Visible")
            w286 = FALSE ("Visible")
            n183 = property on="Test Slider" class="Slide (strict)"("Visible"=w287) -> ()  [unwired: 2 in, 2 out]
            n184 = property on="On/Off" class="Bool (strict)"("Visible"=w287) -> ()  [unwired: 2 in, 2 out]
            n185 = property on="Rev/Fwd" class="Clust (strict)"("Visible"=w287) -> ()  [unwired: 2 in, 2 out]
            n186 = property on="Test Ring" class="Ring (strict)"("Visible"=w286) -> ()  [unwired: 2 in, 2 out]
            n187 = property on="Motor" class="Clust (strict)"("Visible"=w286) -> ()  [unwired: 2 in, 2 out]
          }
          frame "Analog Out", "Motor", "PWM" {
            w293 = FALSE ("Visible")
            n188 = case shown="\"Analog Out\"" w292 {
              tunnel: [1.0 ("Value") -1.0 ("Value") 0.0 ("Value")] -> w291
              tunnel: [255.0 ("Value") 1.0 ("Value") 5.0 ("Value")] -> w290
              tunnel: [128.0 ("Value") 0.0 ("Value") 0.0 ("Value")] -> w289
              tunnel: [64.0 ("Value") 0.5 ("Value") 1.0 ("Value")] -> w288
              frame "PWM" {
              }
              frame "Motor", Default {
              }
              frame "Analog Out" {
              }
            }
            n189 = property on="Test Slider" class="Slide (strict)"("Visible"=w293) -> ()  [unwired: 2 in, 2 out]
            n190 = property on="Test Ring" class="Ring (strict)"("Visible"=w293) -> ()  [unwired: 2 in, 2 out]
            n191 = property on="On/Off" class="Bool (strict)"("Visible"=w293) -> ()  [unwired: 2 in, 2 out]
            n192 = property on="Rev/Fwd" class="Clust (strict)"("Visible"=w293) -> ()  [unwired: 2 in, 2 out]
            n193 = property on="Motor" class="Clust (strict)"("Visible"=TRUE) -> ()  [unwired: 2 in, 2 out]
            n194 = property on="Value" class="Slide (strict)"("Value"=w289, "Scale.Minimum"=w291, "Scale.Maximum"=w290, "Scale.Increment"=w288) -> ()  [unwired: 2 in, 2 out]
          }
          frame "Servo" {
            w309 = FALSE ("Visible")
            n195 = call <vilib>:"NT Read Number.vi"("Name"=w311) -> ("Numeric"=w310:dbl)  [unwired: 9 in, 1 out]
            n196 = property on="Motor" class="Clust (strict)"("Visible"=w309) -> ()  [unwired: 2 in, 2 out]
            n197 = property on="Test Ring" class="Ring (strict)"("Visible"=w309) -> ()  [unwired: 2 in, 2 out]
            n198 = property on="On/Off" class="Bool (strict)"("Visible"=w309) -> ()  [unwired: 2 in, 2 out]
            n199 = property on="Rev/Fwd" class="Clust (strict)"("Visible"=w309) -> ()  [unwired: 2 in, 2 out]
            n200 = property on="Test Slider" class="Slide (strict)"("Visible"=TRUE, "Scale.Maximum"=170.0 ("Scale.Range:Maximum")) -> ()  [unwired: 2 in, 2 out]
            n201 = local write "Test Slider"(w310) -> ()
          }
          frame "Relay", "Solenoid" {
            w312 = FALSE ("Visible")
            n202 = property on="Motor" class="Clust (strict)"("Visible"=w312) -> ()  [unwired: 2 in, 2 out]
            n203 = property on="Test Slider" class="Slide (strict)"("Visible"=w312) -> ()  [unwired: 2 in, 2 out]
            n204 = property on="Test Ring" class="Ring (strict)"("Visible"=w312) -> ()  [unwired: 2 in, 2 out]
            n205 = Search and Replace String(input string=w313, search string="/Value  **", replace string="/Direction") -> (result string=w319:string)  [unwired: 5 in, 3 out]
            n206 = call <vilib>:"NT Read String.vi"("Name"=w319) -> ("String"=w317:string)  [unwired: 9 in, 1 out]
            n207 = Equal?(x="Both directions", y=w317) -> (x = y?=w315:bool)
            n208 = property on="Rev/Fwd" class="Clust (strict)"("Visible"=w315) -> ()  [unwired: 2 in, 2 out]
            n209 = Not(x=w315) -> (.not. x?=w316:bool)
            n210 = property on="On/Off" class="Bool (strict)"("Visible"=w316, "Caption.Text"=w314) -> ()  [unwired: 2 in, 2 out]
          }
          frame "Compressor", "Digital Out" {
            w322 = FALSE ("Visible")
            # "Get direction and finish"
            n211 = property on="Test Ring" class="Ring (strict)"("Visible"=w322) -> ()  [unwired: 2 in, 2 out]
            n212 = property on="Motor" class="Clust (strict)"("Visible"=w322) -> ()  [unwired: 2 in, 2 out]
            n213 = property on="Test Slider" class="Slide (strict)"("Visible"=w322) -> ()  [unwired: 2 in, 2 out]
            n214 = property on="Rev/Fwd" class="Clust (strict)"("Visible"=FALSE) -> ()  [unwired: 2 in, 2 out]
            n215 = property on="On/Off" class="Bool (strict)"("Visible"=TRUE, "Caption.Text"=w323) -> ()  [unwired: 2 in, 2 out]
          }
          frame "Camera" {
            n216 = call <vilib>:"Get Last Path Segment.vi"("String in"=w330) -> ("String out"=w331:string)  [unwired: 10 in]
            n217 = property on="On/Off" class="Bool (strict)"("Visible"=FALSE) -> ()  [unwired: 2 in, 2 out]
            n218 = case shown="\"White Balance  **\"" w331 {
              tunnel: w330 -> [w337 w346 w355 w364 w373 _ w379]
              tunnel: w329 -> [w335 w343 w352 w361 w370 _ _]
              frame "Size  **" {
                n219 = Index Array(array=w335) -> (element=w334:cluster{string[]})  [unwired: 1 in]
                n220 = call <vilib>:"NT Read String.vi"("Name"=w337) -> ("String"=w336:string)  [unwired: 9 in, 1 out]
                n221 = property on="Test Slider" class="Slide (strict)"("Visible"=FALSE) -> ()  [unwired: 2 in, 2 out]
                n222 = property on="Test Ring" class="Ring (strict)"("Visible"=TRUE) -> ()  [unwired: 2 in, 2 out]
                n223 = Unbundle(w334) -> (w332:string[])
                n224 = Match First String(2:w332, 3:w336) -> (0:w333:i32)  [unwired: 1 out]
                n225 = property on="Test Ring" class="Ring (strict)"("Value"=w333, "Strings []"=w332) -> ()  [unwired: 2 in, 2 out]
              }
              frame "White Balance  **" {
                n226 = call <vilib>:"NT Read String.vi"("Name"=w346) -> ("String"=w345:string)  [unwired: 9 in, 1 out]
                n227 = Index Array(array=w343, index=1) -> (element=w344:cluster{string[]})
                n228 = property on="Test Slider" class="Slide (strict)"("Visible"=FALSE) -> ()  [unwired: 2 in, 2 out]
                n229 = property on="Test Ring" class="Ring (strict)"("Visible"=TRUE) -> ()  [unwired: 2 in, 2 out]
                n230 = Unbundle(w344) -> (w341:string[])
                n231 = Match First String(2:w341, 3:w345) -> (0:w340:i32)  [unwired: 1 out]
                n232 = property on="Test Ring" class="Ring (strict)"("Value"=w340, "Strings []"=w341) -> ()  [unwired: 2 in, 2 out]
              }
              frame "Exposure  **" {
                n233 = call <vilib>:"NT Read String.vi"("Name"=w355) -> ("String"=w354:string)  [unwired: 9 in, 1 out]
                n234 = Index Array(array=w352, index=2) -> (element=w353:cluster{string[]})
                n235 = property on="Test Slider" class="Slide (strict)"("Visible"=FALSE) -> ()  [unwired: 2 in, 2 out]
                n236 = property on="Test Ring" class="Ring (strict)"("Visible"=TRUE) -> ()  [unwired: 2 in, 2 out]
                n237 = Unbundle(w353) -> (w349:string[])
                n238 = Match First String(2:w349, 3:w354) -> (0:w350:i32)  [unwired: 1 out]
                n239 = property on="Test Ring" class="Ring (strict)"("Value"=w350, "Strings []"=w349) -> ()  [unwired: 2 in, 2 out]
              }
              frame "Exposure Priority  **" {
                n240 = call <vilib>:"NT Read String.vi"("Name"=w364) -> ("String"=w363:string)  [unwired: 9 in, 1 out]
                n241 = Index Array(array=w361, index=3) -> (element=w362:cluster{string[]})
                n242 = property on="Test Slider" class="Slide (strict)"("Visible"=FALSE) -> ()  [unwired: 2 in, 2 out]
                n243 = property on="Test Ring" class="Ring (strict)"("Visible"=TRUE) -> ()  [unwired: 2 in, 2 out]
                n244 = Unbundle(w362) -> (w358:string[])
                n245 = Match First String(2:w358, 3:w363) -> (0:w359:i32)  [unwired: 1 out]
                n246 = property on="Test Ring" class="Ring (strict)"("Value"=w359, "Strings []"=w358) -> ()  [unwired: 2 in, 2 out]
              }
              frame "Color Enable  **" {
                n247 = call <vilib>:"NT Read String.vi"("Name"=w373) -> ("String"=w372:string)  [unwired: 9 in, 1 out]
                n248 = Index Array(array=w370, index=4) -> (element=w371:cluster{string[]})
                n249 = property on="Test Slider" class="Slide (strict)"("Visible"=FALSE) -> ()  [unwired: 2 in, 2 out]
                n250 = property on="Test Ring" class="Ring (strict)"("Visible"=TRUE) -> ()  [unwired: 2 in, 2 out]
                n251 = Unbundle(w371) -> (w367:string[])
                n252 = Match First String(2:w367, 3:w372) -> (0:w368:i32)  [unwired: 1 out]
                n253 = property on="Test Ring" class="Ring (strict)"("Value"=w368, "Strings []"=w367) -> ()  [unwired: 2 in, 2 out]
              }
              frame Default {
                n254 = property on="Test Slider" class="Slide (strict)"("Visible"=FALSE) -> ()  [unwired: 2 in, 2 out]
                n255 = property on="Test Ring" class="Ring (strict)"("Visible"=FALSE) -> ()  [unwired: 2 in, 2 out]
              }
              frame "Brightness  **", "Color Level  **", "Compression  **", "FPS  **", "Sharpness  **" {
                n256 = call <vilib>:"NT Read Number.vi"("Name"=w379) -> ("Numeric"=w378:dbl)  [unwired: 9 in, 1 out]
                n257 = property on="Test Ring" class="Ring (strict)"("Visible"=FALSE) -> ()  [unwired: 2 in, 2 out]
                n258 = property on="Test Slider" class="Slide (strict)"("Visible"=TRUE, "Scale.Maximum"=100.0 ("Scale.Range:Maximum")) -> ()  [unwired: 2 in, 2 out]
                n259 = local write "Test Slider"(w378) -> ()
              }
            }
            n260 = property on="Motor" class="Clust (strict)"("Visible"=FALSE) -> ()  [unwired: 2 in, 2 out]
            n261 = property on="Rev/Fwd" class="Clust (strict)"("Visible"=FALSE) -> ()  [unwired: 2 in, 2 out]
          }
        }
      }
      event "Test Name": Mouse Enter {
        # "Populate the ring with the list of tests"
        n262 = event-data() -> ()  [unwired: 1 in, 1 out]
        n263 = call <vilib>:"NT Read String Array.vi"("Name"="/TestMode/TestList") -> ("String Array"=w388:string[])  [unwired: 9 in, 1 out]
        n264 = Build Array (concatenate)("Select the test to run...", w388) -> (w387:string[])
        n265 = property on="Test Name" class="Ring (strict)"("Strings []"=w387) -> ()  [unwired: 2 in, 2 out]
      }
      event "Test Name": Value Change {
        w391 = FALSE ("Visible")
        # "Tell the robot the test name to run"
        n266 = event-data() -> ("NewVal"=w395:u16)  [unwired: 1 in]
        n267 = property on="Test Name" class="Ring (strict)"() -> ("Strings []"=w396:string[])  [unwired: 2 in, 2 out]
        n268 = property on="Test Ring" class="Ring (strict)"("Visible"=w391) -> ()  [unwired: 2 in, 2 out]
        n269 = property on="Motor" class="Clust (strict)"("Visible"=w391) -> ()  [unwired: 2 in, 2 out]
        n270 = property on="Test Slider" class="Slide (strict)"("Visible"=w391) -> ()  [unwired: 2 in, 2 out]
        n271 = property on="On/Off" class="Bool (strict)"("Visible"=w391) -> ()  [unwired: 2 in, 2 out]
        n272 = property on="Rev/Fwd" class="Clust (strict)"("Visible"=w391) -> ()  [unwired: 2 in, 2 out]
        n273 = property on="Progress" class="Clust (strict)"("Visible"=TRUE) -> ()  [unwired: 2 in, 2 out]
        n274 = local write "Progress"(T7 {"Test Progress"=0, "Test Progress Text"=""} ("Progress")) -> ()
        n275 = Index Array(array=w396, index=w395) -> (element=w394:string)
        n276 = call <vilib>:"NT Write String.vi"("String"=w394, "Name"="/TestMode/TestName") -> ()  [unwired: 9 in, 1 out]
      }
      event "Select Auto": Mouse Enter {
        # "Populate the combo box with the list of autonomous options"
        n277 = event-data() -> ()  [unwired: 1 in, 1 out]
        n278 = call <vilib>:"NT Read String Array.vi"("Name"="Auto List") -> ("String Array"=w398:string[])  [unwired: 9 in, 1 out]
        n279 = property on="Select Auto" class="CmbBox"("Strings[]"=w398) -> ()  [unwired: 2 in, 2 out]
      }
      event "Select Auto": Value Change {
        # "User modified the Auto Selection. Write to NT variable so robot knows."
        n280 = event-data() -> ("NewVal"=w402:string)  [unwired: 1 in]
        n281 = call <vilib>:"NT Write String.vi"("String"=w402, "Name"="Auto Selector") -> ()  [unwired: 9 in, 1 out]
      }
      event "Command Selection": Value Change {
        # "Get the params and show in table"
        n282 = event-data() -> ("NewVal"=w409:i32)  [unwired: 1 in]
        n283 = property on="Command Selection" class="MCListbox (strict)"() -> ("ItemNames"=w407:string[][])  [unwired: 2 in, 2 out]
        n284 = call <vilib>:"WPI_DashboardUpdate Command Params.vi"("NewVal"=w409, "Commands"=w407, "Param Tbl"=w408) -> ()  [unwired: 8 in, 1 out]
      }
      event "Execute Command": Value Change {
        # "Started one, Unique ID holds\nresponse"
        n285 = event-data() -> ()  [unwired: 1 in, 1 out]
        n286 = property on="Command Selection" class="MCListbox (strict)"() -> ("ItemNames"=w421:string[][])  [unwired: 2 in, 2 out]
        n287 = Index Array(array=w421, index (row)="Command Selection", index (col)=0) -> (element=w419:string)
        n288 = call <vilib>:"Invoke Commands.vi"("Command Params"="Command Params", "Function Name"=w419) -> ("Params"=w415:u8, "Started"=w414:bool)  [unwired: 7 in, 1 out]
        n289 = Array Subset(array="Command Params", length (row)=w415) -> (w416:string[][])  [unwired: 3 in]
        n290 = Select(t="Executing" ("Cmd Status"), s=w414, f="" ("Cmd Status")) -> (s? t:f=→"Cmd Status":string)
      }
      event "Command Selection": Double Click {
        n291 = event-data() -> ("Row"=w431:i32)  [unwired: 1 in]
        n292 = property on="Command Selection" class="MCListbox (strict)"() -> ("ItemNames"=w434:string[][])  [unwired: 2 in, 2 out]
        n293 = local read "Command Params"() -> (w429:string[][])
        n294 = Index Array(array=w434, index (row)=w431, index (col)=0) -> (element=w432:string)
        n295 = call <vilib>:"Invoke Commands.vi"("Command Params"=w429, "Function Name"=w432) -> ("Params"=w428:u8, "Started"=w423:bool)  [unwired: 7 in, 1 out]
        n296 = Array Subset(array=w429, length (row)=w428) -> (w427:string[][])  [unwired: 3 in]
        n297 = Select(t="Executing" ("Cmd Status"), s=w423, f="" ("Cmd Status")) -> (s? t:f=w424:string)
        n298 = local write "Cmd Status"(w424) -> ()
      }
      event "CheckList": Double Click {
        # "Shift clears all"
        # "Update symbols on the listbox"
        n299 = event-data() -> ("PlatMods.Shift"=w437:bool, "Row"=w439:i32)  [unwired: 1 in]
        n300 = case shown="True" w437 {
          tunnel: w439 -> [w443 _]
          tunnel: 1 -> [w442 _]
          frame False {
            n301 = property on="CheckList" class="LstBox (strict)"() -> ("Item Symbols"=w441:i32[])  [unwired: 2 in, 2 out]
            n302 = Replace Array Subset(array=w441, new element=w442, index=w443) -> (w440:i32[])
            n303 = property on="CheckList" class="LstBox (strict)"("Item Symbols"=w440) -> ()  [unwired: 2 in, 2 out]
          }
          frame True {
            w444 = 0 ("Top Row")
            n304 = property on="CheckList" class="LstBox (strict)"() -> ("Number of Rows"=w446:u32)  [unwired: 2 in, 2 out]
            n305 = Initialize Array(0, w446) -> (w445:i32[])
            n306 = property on="CheckList" class="LstBox (strict)"("Top Row"=w444, "Value"=w444, "Item Symbols"=w445) -> ()  [unwired: 2 in, 2 out]
          }
        }
      }
      event "CheckList": Key Down {
        # "Update symbols on the listbox\nLeft and right keys check and uncheck"
        n307 = event-data() -> ("VKey"=w451:T29)  [unwired: 1 in]
        n308 = case shown="\"Left\", \"Right\"" w451 {
          selector: w451 -> [w456 _]
          tunnel: eventvkey."Left" ("VKey") -> [w454 _]
          frame "Left", "Right" {
            n309 = Equal?(x=w454, y=w456) -> (x = y?=w455:bool)
            n310 = Select(t=0, s=w455, f=1) -> (s? t:f=w457:i32)
            n311 = property on="CheckList" class="LstBox (strict)"() -> ("Item Symbols"=w460:i32[])  [unwired: 2 in, 2 out]
            n312 = Replace Array Subset(array=w460, new element=w457, index="CheckList") -> (w459:i32[])
            n313 = property on="CheckList" class="LstBox (strict)"("Item Symbols"=w459) -> ()  [unwired: 2 in, 2 out]
          }
          frame Default {
          }
        }
      }
      event "DB Camera Config": Value Change {
        # "Show or hide the cluster of controls, store in ini file"
        n314 = event-data() -> ("NewVal"=w465:bool)  [unwired: 1 in]
        n315 = case shown="False" w465 {
          tunnel: w464 -> [w474 _]
          tunnel: [w467 w485] -> w463
          tunnel: w462 -> [w466 w485]
          frame False {
            w481 = "Camera"
            w484 = FALSE ("Visible")
            n316 = Index Array(array=w474) -> (element=w477:cluster{string[]})  [unwired: 1 in]
            n317 = property on="Camera Settings" class="Clust (strict)"("Visible"=w484) -> ()  [unwired: 2 in, 2 out]
            n318 = local write "DB Camera Config"(w484) -> ()
            n319 = Unbundle(w477) -> (w476:string[])
            n320 = local read "Camera Settings"() -> (w473:T2)
            n321 = Unbundle(w473) -> ("Frame Rate"=w472:i32, "Compression"=w471:i32, "Size"=w475:u16)
            n322 = Index Array(array=w476, index=w475) -> (element=w470:string)
            n323 = call-poly <vilib>:"Write Key.vi"("section"=w481, "value"=w470, "key"="Size", "refnum"=w466) -> ("refnum out"=w483:T27)  [unwired: 2 in, 5 out]
            n324 = call-poly <vilib>:"Write Key.vi"("section"=w481, "value"=w472, "key"="FrameRate", "refnum"=w483) -> ("refnum out"=w482:T27)  [unwired: 1 in, 6 out]
            n325 = call-poly <vilib>:"Write Key.vi"("section"=w481, "value"=w471, "key"="Compression", "refnum"=w482) -> ("refnum out"=w468:T27)  [unwired: 1 in, 6 out]
            n326 = call <vilib>:"Close Config Data.vi"("refnum"=w468) -> ("file path"=w469:path)  [unwired: 2 in, 8 out]
            n327 = call <vilib>:"Open Config Data.vi"("configuration file path"=w469) -> ("refnum"=w467:T27)  [unwired: 8 in, 2 out]
          }
          frame True {
            n328 = property on="Camera Settings" class="Clust (strict)"("Visible"=TRUE) -> ()  [unwired: 2 in, 2 out]
          }
        }
      }
      event "Camera Settings": Value Change {
        # "Update summary string when any elements of DB camera change"
        n329 = event-data() -> ("NewVal"=w499:T2)  [unwired: 1 in]
        n330 = Index Array(array=w495) -> (element=w494:cluster{string[]})  [unwired: 1 in]
        n331 = Unbundle(w499) -> ("Frame Rate"=w490:i32, "Compression"=w489:i32, "Size"=w492:u16)
        n332 = Unbundle(w494) -> (w493:string[])
        n333 = Index Array(array=w493, index=w492) -> (element=w491:string)
        n334 = Format Into String(format string="%s   %dfps   %d%%", w491, w490, w489) -> (resulting string=w496:string)  [unwired: 2 in, 1 out]
        n335 = Build Array(w496) -> (w497:string[])
        n336 = property on="DB Camera Config" class="Bool (strict)"("Strings [4]"=w497) -> ()  [unwired: 2 in, 2 out]
      }
      event "Motor.Enable": Value Change {
        # "When the test mode otor enable helper is set, update that\ntree row item's value"
        n337 = event-data() -> ("NewVal"=w506:bool)  [unwired: 1 in]
        n338 = Unbundle("Motor") -> ("Value"=w505:dbl)  [unwired: 1 out]
        n339 = Select(t=w505, s=w506, f=0.0) -> (s? t:f=w503:dbl)
        n340 = call <vilib>:"NT Write Number.vi"("Numeric"=w503, "Name"=w502) -> ()  [unwired: 9 in, 1 out]
      }
      event "Test Slider": Value Change {
        # "When the test mode slider helper is set, update that\ntree row item's value"
        n341 = event-data() -> ("NewVal"=w510:dbl)  [unwired: 1 in]
        n342 = call <vilib>:"NT Write Number.vi"("Numeric"=w510, "Name"=w511) -> ()  [unwired: 9 in, 1 out]
      }
      event "On/Off": Value Change {
        # "When the test mode on/off helper value is set, update that\ntree row item's value"
        n343 = event-data() -> ("NewVal"=w516:bool)  [unwired: 1 in]
        n344 = Boolean To (0,1)(Boolean=w516) -> (0, 1=w515:i16)
        n345 = call <vilib>:"NT Write Number.vi"("Numeric"=w515, "Name"=w514) -> ()  [unwired: 9 in, 1 out]
      }
      event "Rev/Fwd": Value Change {
        # "When the test mode helper value for relays is set, update that\ntree row item's value"
        n346 = event-data() -> ("NewVal.Forward"=w525:bool, "NewVal.Reverse"=w524:bool)  [unwired: 1 in]
        n347 = Boolean To (0,1)(Boolean=w525) -> (0, 1=w521:i16)
        n348 = Boolean To (0,1)(Boolean=w524) -> (0, 1=w523:i16)
        n349 = Negate(x=w523) -> (-x=w522:i16)
        n350 = Add(x=w521, y=w522) -> (x+y=w520:i16)
        n351 = call <vilib>:"NT Write Number.vi"("Numeric"=w520, "Name"=w519) -> ()  [unwired: 9 in, 1 out]
      }
      event "Test Ring": Value Change {
        # "When a test mode helper value is selected from the ring,\nset the tree item's variable to the string value"
        n352 = event-data() -> ("NewVal"=w530:u16)  [unwired: 1 in]
        n353 = property on="Test Ring" class="Ring (strict)"() -> ("Strings []"=w531:string[])  [unwired: 2 in, 2 out]
        n354 = Index Array(array=w531, index=w530) -> (element=w529:string)
        n355 = call <vilib>:"NT Write String.vi"("String"=w529, "Name"=w528) -> ()  [unwired: 9 in, 1 out]
      }
      event "Rec Mode": Value Change {
        # "Update globals for recording mode and path to read log from.\nClear when logging and let NetworkTables set path for vision to\nuse."
        n356 = event-data() -> ("NewVal"=w543:enum32{"Stop", "Record", "Playback"})  [unwired: 1 in]
        n357 = global write "WPI_DashboardLogging Global.vi" "Logging Filename"(path "") -> ()
        n358 = global write "WPI_DashboardLogging Global.vi" "Recording"(w543) -> ()
        n359 = case shown="\"Playback\"" w543 {
          tunnel: w542 -> [_ w545 w554]
          tunnel: [_ _ w553] -> w539
          tunnel: [_ _ w552] -> _
          tunnel: w537 -> [_ _ w550]
          tunnel: cluster{i32, i32} {-250, 170} -> [_ _ w549]
          tunnel: [_ _ T30 {"Image Size"=TRUE, "Image Type"=TRUE, "Pixel Value"=TRUE, "ROI Information"=TRUE, "Zoom Factor"=FALSE} ("Image Information Shown:All Elements")] -> w535
          tunnel: [_ _ TRUE ("Zoom Factor")] -> w534
          tunnel: w533 -> [_ _ w546]
          frame Default {
          }
          frame "Stop", "Record" {
            # "Place Window too"
            n360 = invoke class="VI" method="FP.Close"(reference=w545) -> (reference out=w544:refnum<vi>)  [unwired: 2 in, 2 out]
            n361 = invoke class="VI" method="Abort VI"(reference=w544) -> ()  [unwired: 2 in, 3 out]
          }
          frame "Playback" {
            n362 = call "Open Playback Panel.vi"("Offset"=w549, "DB VI Ref"=w550, "Playback in"=w554) -> ("Playback out"=w551:refnum<vi>)  [unwired: 8 in]
            n363 = register-events(w551, w546) -> (reference out=w553:refnum<event-registration>, error out=w552:errorcluster)  [unwired: 2 in]
          }
        }
        n364 = property on="Camera Image" class="ImageControl"("Image Information Shown"=w535, "Image Information Visible"=w534) -> ()  [unwired: 2 in, 2 out]
        n365 = call <vilib>:"WPI_DashboardNT Log FieldName Cache.vi"("Operation"=enum16{"Lookup/Add", "Index", "Clear"}."Clear") -> ()  [unwired: 8 in, 3 out]
      }
      event Panel Close {
        w556 = enum32{"Stop", "Record", "Playback"}."Stop" ("Rec Mode")
        # "Playback window has been closed, abort"
        n366 = event-data() -> ()  [unwired: 1 in, 4 out]
        n367 = local write "Rec Mode"(w556) -> ()
        n368 = global write "WPI_DashboardLogging Global.vi" "Recording"(w556) -> ()
      }
      event Panel Close {
        # "Abort playback window and ourself"
        n369 = event-data() -> ()  [unwired: 1 in, 4 out]
        n370 = invoke class="VI" method="FP.Close"(reference=w562) -> (reference out=w561:refnum<vi>)  [unwired: 2 in, 2 out]
        n371 = invoke class="VI" method="Abort VI"(reference=w561) -> (error out=w560:errorcluster)  [unwired: 2 in, 2 out]
        n372 = invoke class="VI" method="Abort VI"(error in=w560) -> ()  [unwired: 2 in, 3 out]
      }
      event User Event {
        n373 = event-data() -> ("IDs"=w570:cluster{"RPC field ID":u16, "Unique ID":u16}, "String"=w569:string)  [unwired: 1 in]
        n374 = local write "Cmd Status"("" ("Cmd Status")) -> ()
        n375 = Bundle("IDs"=w570, "String"=w569) -> (w568:T16)  [unwired: 1 in]
        n376 = call <vilib>:"Retrieve RPC Response.vi"("RPC Response"=w568) -> ("Output"=w565:string[][])  [unwired: 10 in]
        n377 = Build Array (concatenate)(w563, w565) -> (w564:string[][])
        n378 = local write "Command Params"(w564) -> ()
      }
      event "Vision": Value Change {
        # "Enable/Disable Compression slider.\nHW USB is hard-coded into the camera"
        n379 = event-data() -> ("NewVal"=w577:u16)  [unwired: 1 in]
        n380 = Equal?(x=w577, y=u32 2 ("milliseconds to wait")) -> (x = y?=w575:bool)
        n381 = Select(t=T31."Disabled and Grayed Out" ("Disabled"), s=w575, f=T31."Enabled" ("Disabled")) -> (s? t:f=w572:T31)
        n382 = property on="Compression" class="Slide (strict)"("DisabledEnum"=w572) -> ()  [unwired: 2 in, 2 out]
      }
      event "Tree": Double Click {
        n383 = event-data() -> ("PlatMods"=w582:T34, "Tag"=w581:string)  [unwired: 1 in]
        n384 = Unbundle(w582) -> ("Shift"=w580:bool)  [unwired: 4 out]
        n385 = Not(x=w580) -> (.not. x?=w579:bool)
        n386 = call <vilib>:"NT Update Persistence.vi"("Persistence"=w579, "Name"=w581) -> ()  [unwired: 9 in, 1 out]
      }
    }
  }
  n387 = while {
    tunnel: w114 -> [w586]
    i -> [w589]
    stop <- FALSE stop-if-true
    n388 = Wait (ms)(milliseconds to wait=u32 100) -> ()  [unwired: 1 out]
    n389 = case shown="\"Playback\"" "Rec Mode" {
      tunnel: w589 -> [_ _ w604]
      tunnel: [u32 2829099 ("Base Color") u32 11141120 ("Target Color") w593] -> w585
      frame "Stop", Default {
        # "Reset the color, extra updates don't cost much"
      }
      frame "Record" {
      }
      frame "Playback" {
        # "Playback"
        n390 = Quotient & Remainder(x=w604, y=u32 50 ("milliseconds to wait")) -> (x-y*floor(x/y)=w600:u32)  [unwired: 1 out]
        n391 = Divide(x=w600, y=u32 50 ("milliseconds to wait")) -> (x/y=w597:dbl)
        n392 = Multiply(x=6.283185307179586, y=w597) -> (x*y=w602:dbl)
        n393 = Sine(x=w602) -> (sin(x)=w601:dbl)
        n394 = Absolute Value(x=w601) -> (abs(x)=w594:dbl)
        n395 = call "Interpolate RGB Color.vi"("Proportion"=w594, "Target Color"=u32 30976, "Base Color"=u32 2829099) -> ("Result Color"=w593:u32)  [unwired: 8 in]
      }
    }
    n396 = property class="Pane"(reference=w586, "PaneColor"=w585) -> ()  [unwired: 1 in, 2 out]
  }
  n397 = local write "Dashboard Tab"(T17."Drive" ("Dashboard Tab")) -> ()
  n398 = property on="On/Off" class="Bool (strict)"("Visible"=w82) -> ()  [unwired: 2 in, 2 out]
  n399 = property on="Motor" class="Clust (strict)"("Visible"=w82) -> ()  [unwired: 2 in, 2 out]
  n400 = property on="Progress" class="Clust (strict)"("Visible"=w82) -> ()  [unwired: 2 in, 2 out]
  n401 = property on="Test Ring" class="Ring (strict)"("Visible"=w82) -> ()  [unwired: 2 in, 2 out]
  n402 = property on="Rev/Fwd" class="Clust (strict)"("Visible"=w82) -> ()  [unwired: 2 in, 2 out]
  n403 = property on="Camera Settings" class="Clust (strict)"("Visible"=w82) -> ()  [unwired: 2 in, 2 out]
  n404 = local write "DB Camera Config"(w82) -> ()
  n405 = local write "Command Params"(string[][] [] ("Command Params")) -> ()
  n406 = global write "WPI_DashboardLogging Global.vi" "Recording"(w108) -> ()
  n407 = local write "Rec Mode"(w108) -> ()
  n408 = while {
    tunnel: u16 1741 ("timeout ms (25000)") -> [w606]
    stop <- FALSE stop-if-true
    n409 = TCP Create Listener(10:w606) -> (0:w605:errorcluster, 3:w607:refnum<k5>)  [unwired: 4 in, 1 out]
    n410 = case shown="No Error" w605 {
      selector: w605 -> [w609 _]
      tunnel: w607 -> [w610 _]
      frame No Error {
        n411 = while {
          tunnel: w610 -> [w613]
          tunnel: w609 -> [w612]
          stop <- FALSE stop-if-true
          n412 = TCP Wait On Listener(8:w612, 11:w613) -> (0:w614:errorcluster, 4:w615:refnum<k5>)  [unwired: 2 in, 3 out]
          n413 = local write "TCP"(w615) -> ()
          n414 = case shown="No Error" w614 {
            frame No Error {
            }
            frame Error {
              n415 = Wait (ms)(milliseconds to wait=u32 1000) -> ()  [unwired: 1 out]
            }
          }
        }
      }
      frame Error {
        n416 = Wait (ms)(milliseconds to wait=u32 1000) -> ()  [unwired: 1 out]
      }
    }
  }
  n417 = local write "Command Selection"(u16 0 ("milliseconds to wait")) -> ()
